vi "Set Component Settings.vi"(8 "error in (no error)":errorcluster, 9 "settings id":T1={"plugin"=-1, "thread"=-1, "group"=-1, "transfer"=-1, "channel"=-1}, 10 "component settings":T2[](array[typedef]), 11 "Configuration Session in":refnum<class "Configuration Session.lvclass">) -> (0 "error out":errorcluster, 3 "Configuration Session out":refnum<class "Configuration Session.lvclass">)   [LabVIEW 2017, in "DSF Core.lvlib" / "Configuration Session.lvclass"]
uses:
  Configuration Session.lvclass
  Typedefs/DSF Settings Info.ctl
  Typedefs/DSF Version Info.ctl
  Typedefs/DSF Configuration ID.ctl
  Configuration Session.lvclass/Configuration Session.ctl
  DSF Core.lvlib
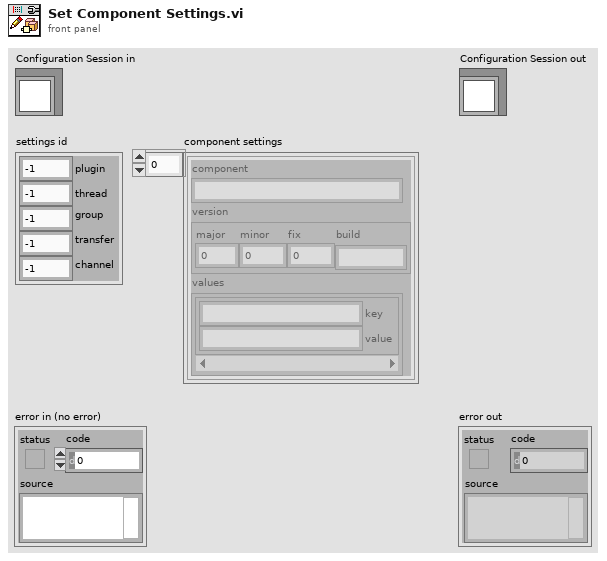
[diagram p1: front panel]
types:
  T1 = typedef "DSF Core.lvlib/DSF Configuration ID.ctl" = cluster{"plugin":i32, "thread":i32, "group":i32, "transfer":i32, "channel":i32}
  T2 = typedef "DSF Core.lvlib/DSF Settings Info.ctl" = cluster{"component":string, "version":T3, "values":cluster{"key":string, "value":string}[]}
  T3 = typedef "DSF Core.lvlib/DSF Version Info.ctl" = cluster{"major":u32, "minor":u32, "fix":u32, "build":string}
  T4 = typedef "DSF Core.lvlib/Configuration Session.lvclass/DSF Config Data Ref.ctl" = refnum<data-value>
  T5 = typedef "DSF Core.lvlib/Configuration Session.lvclass/DSF Config Data.ctl" = cluster{"dsf configuration":T6, "path":path, "dirty":bool}
  T6 = typedef "DSF Core.lvlib/Configuration Session.lvclass/Internal DSF Configuration.ctl" = cluster{"dsfversion":T3, "version":T3, "plugins":T7[], "groups":T21[], "transfers":T23[], "channels":T25[], "settings":T27[], "framework configuration":T29, "configuration":refnum<class>}
  T7 = typedef "DSF Core.lvlib/Configuration Session.lvclass/Internal DSF Plugin with ID.ctl" = cluster{"id":string, "values":T8}
  T8 = typedef "DSF Core.lvlib/Configuration Session.lvclass/Internal DSF Plugin Info.ctl" = cluster{"components":string[], "timing":T9, "group ids":string[], "settings id":string, "threads":T10[]}
  T9 = typedef "DSF Core.lvlib/DSF Timing Info.ctl" = cluster{"priority":u64, "decimation":u64, "offset":u64}
  T10 = typedef "DSF Core.lvlib/DSF Engine Plugin Thread Configuration.ctl" = cluster{"core":T11, "component settings":T2[], "transfer groups":T12[]}
  T11 = typedef "DSF Core.lvlib/DSF Core Thread Configuration.ctl" = cluster{"processor":i32, "priority offset":i16}
  T12 = typedef "DSF Core.lvlib/DSF Engine Transfer Group Configuration.ctl" = cluster{"core":T13, "component settings":T2[], "transfers":T16[]}
  T13 = typedef "DSF Core.lvlib/DSF Core Group Configuration.ctl" = cluster{"name":string, "direction":T14, "cycle timing":T9, "timeout behavior":T15}
  T14 = typedef "DSF Core.lvlib/DSF Direction.ctl" = enum8{"Tx", "Rx"}
  T15 = typedef "DSF Core.lvlib/DSF Timeout Behavior.ctl" = enum8{"Increment Late Count", "Throw Error"}
  T16 = typedef "DSF Core.lvlib/DSF Engine Transfer Configuration.ctl" = cluster{"core":T17, "component settings":T2[], "channels":T18[]}
  T17 = typedef "DSF Core.lvlib/DSF Core Transfer Configuration.ctl" = cluster{"name":string}
  T18 = typedef "DSF Core.lvlib/DSF Engine Channel Configuration.ctl" = cluster{"core":T19, "component settings":T2[]}
  T19 = typedef "DSF Core.lvlib/DSF Core Channel Configuration.ctl" = cluster{"name":string, "units":string, "engine data type":T20, "string data type":T20, "string offset":u64}
  T20 = typedef "DSF Core.lvlib/DSF Data Type.ctl" = enum8{"Bool", "SGL", "DBL", "I8", "I16", "I32", "I64", "U8", "U16", "U32", "U64"}
  T21 = typedef "DSF Core.lvlib/Configuration Session.lvclass/Internal DSF Group with ID.ctl" = cluster{"id":string, "values":T22}
  T22 = typedef "DSF Core.lvlib/Configuration Session.lvclass/Internal DSF Group Info.ctl" = cluster{"direction":i32, "timing":T9, "transfer ids":string[], "settings id":string, "thread":i32, "timeout behavior":u8}
  T23 = typedef "DSF Core.lvlib/Configuration Session.lvclass/Internal DSF Transfer with ID.ctl" = cluster{"id":string, "values":T24}
  T24 = typedef "DSF Core.lvlib/Configuration Session.lvclass/Internal DSF Transfer Info.ctl" = cluster{"byte order":i32, "channel ids":string[], "settings id":string}
  T25 = typedef "DSF Core.lvlib/Configuration Session.lvclass/Internal DSF Channel with ID.ctl" = cluster{"id":string, "values":T26}
  T26 = typedef "DSF Core.lvlib/Configuration Session.lvclass/Internal DSF Channel Info.ctl" = cluster{"string buffer offset":u64, "string data type":i32, "engine data type":i32, "settings id":string, "units":string}
  T27 = typedef "DSF Core.lvlib/Configuration Session.lvclass/Internal DSF Settings with ID.ctl" = cluster{"id":string, "values":T28}
  T28 = typedef "DSF Core.lvlib/Configuration Session.lvclass/Internal DSF Settings Info.ctl" = cluster{"key":string, "value":string}[]
  T29 = typedef "DSF Core.lvlib/DSF Engine Framework Configuration.ctl" = cluster{"plugins":T30[]}
  T30 = typedef "DSF Core.lvlib/DSF Engine Plugin Configuration.ctl" = cluster{"core":T31, "component settings":T2[], "threads":T10[]}
  T31 = typedef "DSF Core.lvlib/DSF Core Plugin Configuration.ctl" = cluster{"name":string, "components":string[], "cycle timing":T9}
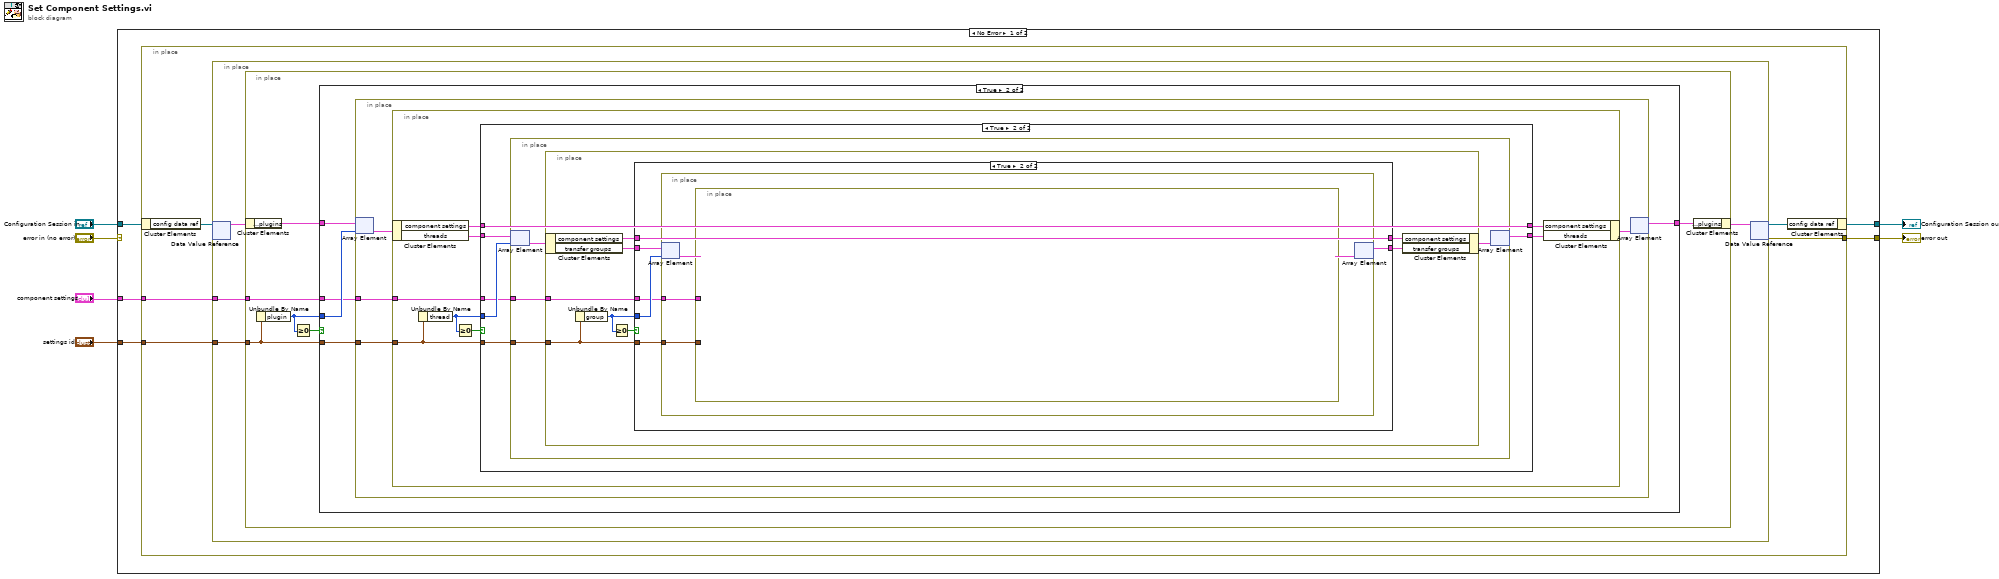
[diagram p0: block diagram]
diagram:
  n1 = case shown="No Error" "error in (no error)" {
    selector: "error in (no error)" -> [_ w115]
    tunnel: [w8 w116] -> w4
    tunnel: "Configuration Session in" -> [w11 w116]
    tunnel: "settings id" -> [w9 _]
    tunnel: [w10 w115] -> w2
    tunnel: "component settings" -> [w7 _]
    frame No Error {
      n2 = in-place {
        in-place-border: [w15] -> w10
        in-place-border: w9 -> [w14]
        in-place-border: w7 -> [w12]
        n3 = in-place-cluster #1(w11) -> ("config data ref"=w16:T4)
        n4 = in-place {
          in-place-border: w14 -> [w20]
          in-place-border: w12 -> [w19]
          n5 = in-place-dvr #2(w16) -> (w18:T5)  [unwired: 1 out]
          n6 = in-place {
            in-place-border: w20 -> [w25]
            in-place-border: w19 -> [w23]
            n7 = in-place-cluster #3(w18) -> ("dsf configuration.framework configuration.plugins"=w22:T30[])
            n8 = Unbundle By Name(w25) -> ("plugin"=w24:i32)
            n9 = Greater Or Equal To 0?(x=w24) -> (x >= 0?=w26:bool)
            n10 = case shown="True" w26 {
              tunnel: w25 -> [_ w32]
              tunnel: w24 -> [_ w30]
              tunnel: w22 -> [w27 w31]
              tunnel: w23 -> [_ w29]
              tunnel: [w27 w28] -> w21
              frame False {
              }
              frame True {
                n11 = in-place {
                  in-place-border: w32 -> [w36]
                  in-place-border: w29 -> [w34]
                  n12 = in-place-array #4(w31, w30) -> (w35:T30)
                  n13 = in-place {
                    in-place-border: w36 -> [w43]
                    in-place-border: w34 -> [w39]
                    n14 = in-place-cluster #5(w35) -> ("component settings"=w40:T2[], "threads"=w41:T10[])
                    n15 = Unbundle By Name(w43) -> ("thread"=w42:i32)
                    n16 = Greater Or Equal To 0?(x=w42) -> (x >= 0?=w44:bool)
                    n17 = case shown="True" w44 {
                      tunnel: w43 -> [_ w52]
                      tunnel: w42 -> [_ w50]
                      tunnel: w41 -> [w46 w51]
                      tunnel: w40 -> [_ w47]
                      tunnel: w39 -> [w45 w49]
                      tunnel: [w46 w48] -> w38
                      tunnel: [w45 w47] -> w37
                      frame False {
                      }
                      frame True {
                        n18 = in-place {
                          in-place-border: w52 -> [w56]
                          in-place-border: w49 -> [w54]
                          n19 = in-place-array #6(w51, w50) -> (w55:T10)
                          n20 = in-place {
                            in-place-border: w56 -> [w64]
                            in-place-border: w54 -> [w59]
                            n21 = in-place-cluster #7(w55) -> ("component settings"=w60:T2[], "transfer groups"=w61:T12[])
                            n22 = Unbundle By Name(w64) -> ("group"=w62:i32)
                            n23 = Greater Or Equal To 0?(x=w62) -> (x >= 0?=w63:bool)
                            n24 = case shown="True" w63 {
                              tunnel: w64 -> [_ w72]
                              tunnel: w62 -> [_ w70]
                              tunnel: w61 -> [w66 w71]
                              tunnel: w60 -> [_ w67]
                              tunnel: w59 -> [w65 w69]
                              tunnel: [w66 w68] -> w58
                              tunnel: [w65 w67] -> w57
                              frame False {
                              }
                              frame True {
                                n25 = in-place {
                                in-place-border: w72 -> [w76]
                                in-place-border: w69 -> [w74]
                                n26 = in-place-array #8(w71, w70) -> (w75:T12)
                                n27 = in-place {
                                in-place-border: w76 -> [w84]
                                in-place-border: w74 -> [w79]
                                n28 = in-place-cluster #9(w75) -> ("component settings"=w81:T2[], "transfers"=w80:T16[])
                                n29 = Unbundle By Name(w84) -> ("transfer"=w82:i32)
                                n30 = Greater Or Equal To 0?(x=w82) -> (x >= 0?=w83:bool)
                                n31 = case shown="True" w83 {
                                tunnel: w84 -> [_ w92]
                                tunnel: w82 -> [_ w91]
                                tunnel: w81 -> [_ w87]
                                tunnel: w80 -> [w86 w90]
                                tunnel: w79 -> [w85 w89]
                                tunnel: [w86 w88] -> w78
                                tunnel: [w85 w87] -> w77
                                frame False {
                                }
                                frame True {
                                n32 = in-place {
                                in-place-border: w92 -> [w96]
                                in-place-border: w89 -> [w94]
                                n33 = in-place-array #10(w90, w91) -> (w95:T16)
                                n34 = in-place {
                                in-place-border: w96 -> [w104]
                                in-place-border: w94 -> [w99]
                                n35 = in-place-cluster #11(w95) -> ("component settings"=w100:T2[], "channels"=w101:T18[])
                                n36 = Unbundle By Name(w104) -> ("channel"=w102:i32)
                                n37 = Greater Or Equal To 0?(x=w102) -> (x >= 0?=w103:bool)
                                n38 = case shown="True" w103 {
                                tunnel: w102 -> [_ w110]
                                tunnel: w101 -> [w106 w111]
                                tunnel: w100 -> [_ w107]
                                tunnel: w99 -> [w105 w109]
                                tunnel: [w106 w108] -> w98
                                tunnel: [w105 w107] -> w97
                                frame False {
                                }
                                frame True {
                                n39 = in-place {
                                in-place-border: w109 -> [w112]
                                n40 = in-place-array #12(w111, w110) -> (w114:T18)
                                n41 = Bundle By Name(cluster=w114, "component settings"=w112) -> (w113:T18)
                                n42 = in-place-array #12(w113) -> (w108:T18[])  [unwired: 1 out]
                                }
                                }
                                }
                                n43 = in-place-cluster #11("component settings"=w97, "channels"=w98) -> (w93:T16)
                                }
                                n44 = in-place-array #10(w93) -> (w88:T16[])  [unwired: 1 out]
                                }
                                }
                                }
                                n45 = in-place-cluster #9("component settings"=w77, "transfers"=w78) -> (w73:T12)
                                }
                                n46 = in-place-array #8(w73) -> (w68:T12[])  [unwired: 1 out]
                                }
                              }
                            }
                            n47 = in-place-cluster #7("component settings"=w57, "transfer groups"=w58) -> (w53:T10)
                          }
                          n48 = in-place-array #6(w53) -> (w48:T10[])  [unwired: 1 out]
                        }
                      }
                    }
                    n49 = in-place-cluster #5("component settings"=w37, "threads"=w38) -> (w33:T30)
                  }
                  n50 = in-place-array #4(w33) -> (w28:T30[])  [unwired: 1 out]
                }
              }
            }
            n51 = in-place-cluster #3("dsf configuration.framework configuration.plugins"=w21) -> (w17:T5)
          }
          n52 = in-place-dvr #2(w17) -> (w13:T4, w15:errorcluster)
        }
        n53 = in-place-cluster #1("config data ref"=w13) -> (w8:refnum<class "Configuration Session.lvclass">)
      }
    }
    frame Error {
    }
  }
  "error out" <- w2
  "Configuration Session out" <- w4
